vi "Plugin - Splash.vi"(11 "Message Queues in":T1) -> ()   [LabVIEW 2019]
uses:
  support/Copy of Message Queue/All Message Queues.ctl
  support/Copy of Message Queue/Message Cluster.ctl
  support/Message Queue/Message Queue.lvlib
  support/Copy of Message Queue/Copy of Message Queue.lvlib
panel:
  in  "error in":errorcluster
  out "error out":errorcluster
  in  "New Calibration":bool
  in  "Exit":bool
  # "Aquatrak Calibration Software\nTransducer Model: 3003-XCR-4"
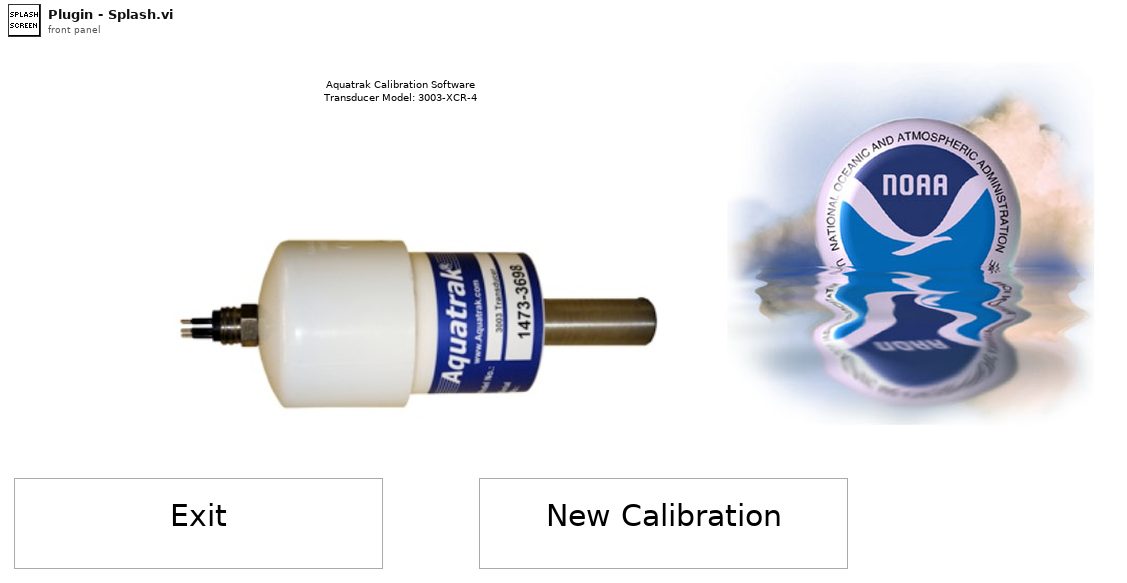
[diagram p1: front panel]
types:
  T1 = typedef "Copy of Message Queue.lvlib/All Message Queues.ctl" = cluster{"UI":refnum<queue>, "Acquisition":refnum<queue>, "Logging":refnum<queue>, "Analyze":refnum<queue>}
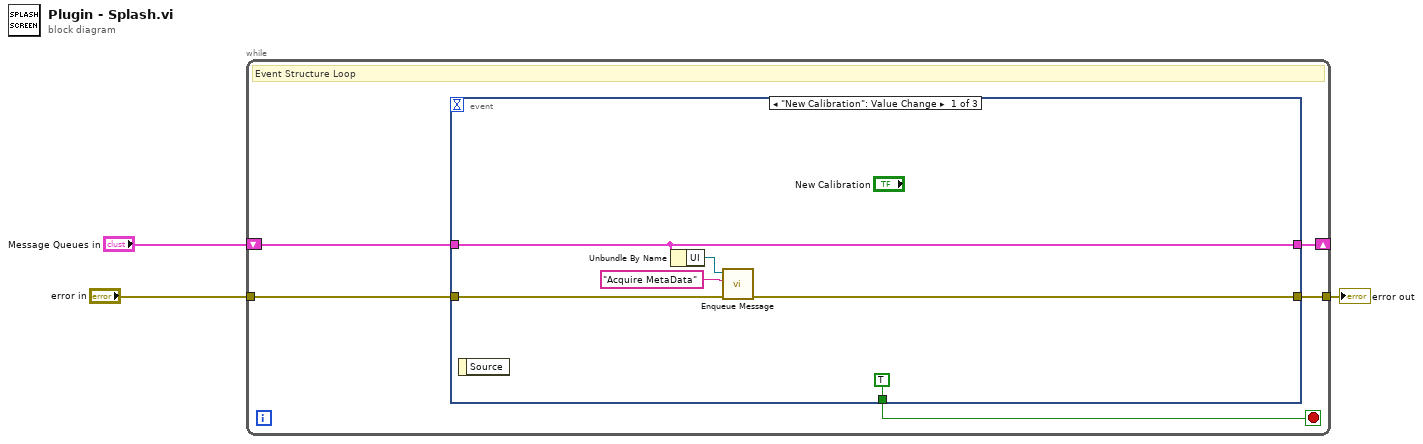
[diagram p0: block diagram]
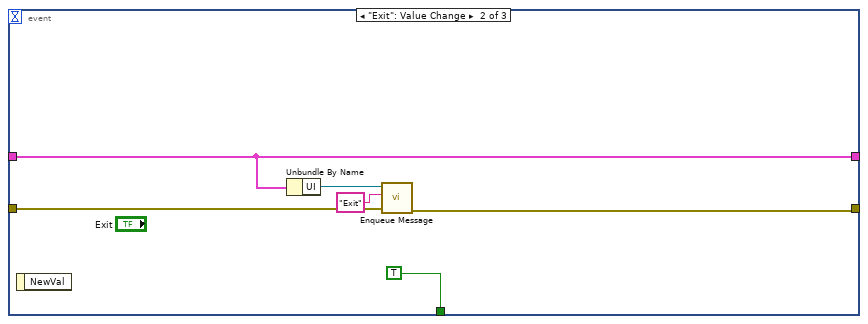
[diagram p2: hidden frame]
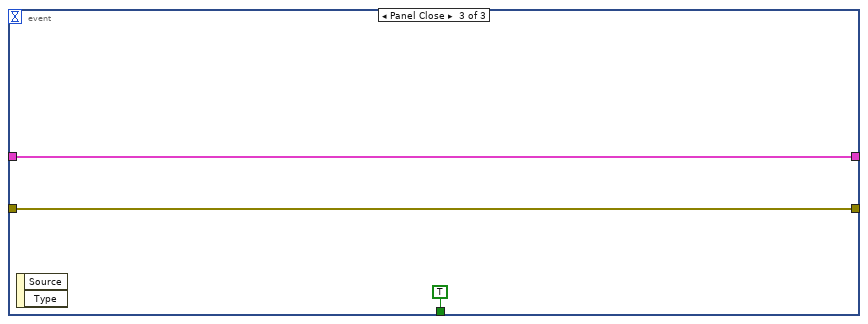
[diagram p3: hidden frame]
diagram:
  n1 = while {
    shift-right: [w7] -> _
    shift-left: "Message Queues in" -> [w6]
    tunnel: [w5] -> w2
    tunnel: "error in" -> [w4]
    stop <- w8 stop-if-true
    # "Event Structure Loop"
    n2 = event shown="[0] \"New Calibration\": Value Change" {
      selector: _ -> [_ _ _]
      dyn-events: _ -> [_ _ _]
      timeout: _ -> [_ _ _]
      tunnel: [TRUE ("NewVal") TRUE ("NewVal") TRUE ("NewVal")] -> w8
      tunnel: w6 -> [w14 w17 w23]
      tunnel: [w14 w17 w23] -> w7
      tunnel: [w10 w15 w21] -> w5
      tunnel: w4 -> [w9 w16 w21]
      event "New Calibration": Value Change {
        n3 = event-data() -> ()  [unwired: 1 in, 1 out]
        n4 = Unbundle By Name(w14) -> ("UI"=w12:refnum<queue>)
        n5 = call "Enqueue Message.vi"("error in (no error)"=w9, "Message"="Acquire MetaData", "Message Queue"=w12) -> ("error out"=w10:errorcluster)  [unwired: 7 in, 1 out]
      }
      event "Exit": Value Change {
        n6 = event-data() -> ()  [unwired: 1 in, 1 out]
        n7 = Unbundle By Name(w17) -> ("UI"=w18:refnum<queue>)
        n8 = call "Enqueue Message.vi"("error in (no error)"=w16, "Message"="Exit", "Message Queue"=w18) -> ("error out"=w15:errorcluster)  [unwired: 7 in, 1 out]
      }
      event Panel Close {
        n9 = event-data() -> ()  [unwired: 1 in, 2 out]
      }
    }
  }
  "error out" <- w2
